vi "Obtain Broadcast Events for Registration.vi"(8 "error in":errorcluster) -> (0 "error out":errorcluster, 2 "Already running?":bool, 3 "Sequence Engine Broadcast Events":T1)   [LabVIEW 2021, in "Sequence Engine.lvlib"]
doc: "Return the broadcast event refnums so the module's caller can register for the module's broadcast events.\n_____\nBased on DQMH Dev Tools: Project Template 7.1.1.1528."
uses:
  Sequence Engine.lvlib
  Broadcast Events--cluster.ctl
  Did Init Argument--cluster.ctl
  Status Updated Argument--cluster.ctl
  Error Reported Argument--cluster.ctl
  Stop Argument--cluster.ctl
  Get Module Execution Status Argument--cluster.ctl
  New Test Result Argument--cluster.ctl
  Classes/Test Result/Result Data.ctl
  Classes/Test Result/Test Status.ctl
  Testing Started Argument--cluster.ctl
  Testing Completed Argument--cluster.ctl
  Retried Count Argument--cluster.ctl
  DUT Info Argument--cluster.ctl
  DUT Info.ctl
  Classes/Test Result/Test Result.lvclass
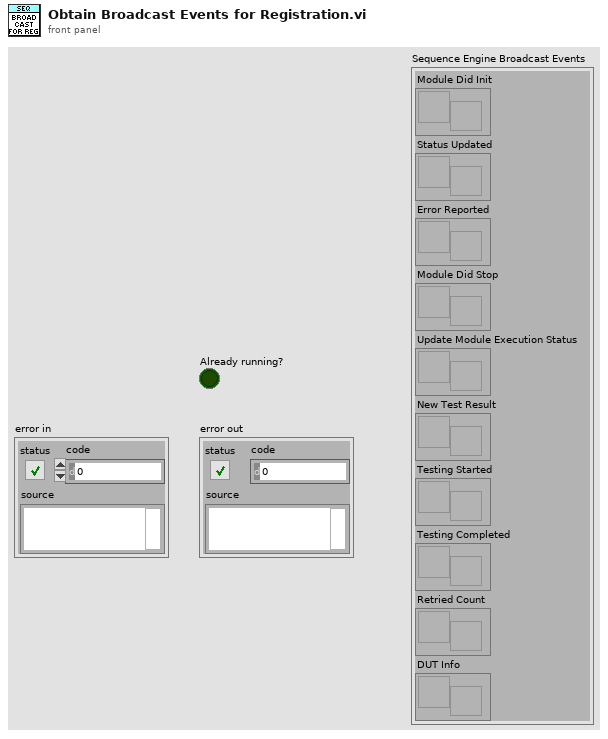
[diagram p1: front panel]
types:
  T1 = typedef "Sequence Engine.lvlib/Broadcast Events--cluster.ctl" = cluster{"Module Did Init":refnum<user-event>, "Status Updated":refnum<user-event>, "Error Reported":refnum<user-event>, "Module Did Stop":refnum<user-event>, "Update Module Execution Status":refnum<user-event>, "New Test Result":refnum<user-event>, "Testing Started":refnum<user-event>, "Testing Completed":refnum<user-event>, "Retried Count":refnum<user-event>, "DUT Info":refnum<user-event>}
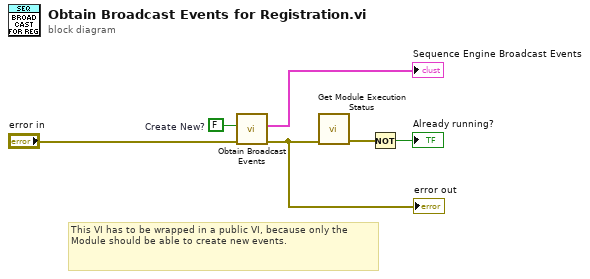
[diagram p0: block diagram]
diagram:
  w5 = FALSE  # Create New?
  # "This VI has to be wrapped in a public VI, because only the Module should be able to create new events."
  n1 = call "Obtain Broadcast Events.vi"("error in"="error in", "Create New? (F)"=w5) -> ("error out"=w4:errorcluster, "Sequence Engine Broadcast Events"=→"Sequence Engine Broadcast Events":T1)  [unwired: 8 in]
  "error out" <- w4
  n2 = call "Get Module Execution Status.vi"("error in"=w4) -> ("error out"=w3:errorcluster)  [unwired: 10 in]
  n3 = Not(x=w3) -> (.not. x?=→"Already running?":bool)
